vi "GlobalVars.vi"() -> ()   [LabVIEW 2015]
uses:
  <vilib>/Rock Robotics/WPI/DriverStation/WPI_DriverStationRobotMode2.ctl
panel:
  out "Robot Mode":T1=enum."Autonomous Enabled"
  out "Number Of Particles":i32
  out "TargetDistance":dbl
  out "LastRememberedX":dbl
  out "DegPerPix":dbl
  out "TargetRight":bool
  out "TargetLeft":bool
  out "OnTarget":bool
  out "RoboRIO IP":string="10.1.95.22"
  out "DesiredGyroValue":dbl
  out "CurrentGyroValue":dbl
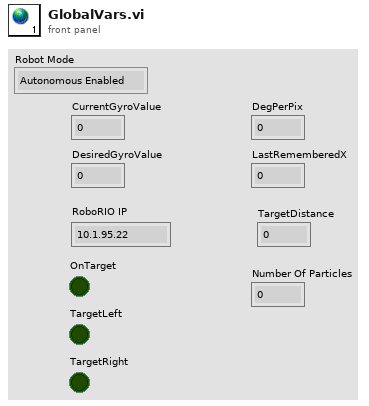
[diagram p1: front panel]
types:
  T1 = typedef "WPI_DriverStationRobotMode2.ctl" = enum16{"Autonomous Disabled", "Autonomous Enabled", "Teleop Disabled", "Teleop Enabled", "Disconnected", "Finish", "Test Disabled", "Test Enabled", "Emergency Stopped"}
diagram:
